vi "Sequence Init.vi"(8 "error in (no error)":errorcluster, 11 "CAP-USB-1 in":refnum<class "CAP-USB-1.lvclass">) -> (0 "error out":errorcluster, 3 "CAP-USB-1 out":refnum<class "CAP-USB-1.lvclass">)   [LabVIEW 2014, in "CAP-USB-1.lvlib" / "CAP-USB-1.lvclass"]
doc: "Envia el codigo de inicializacion para el funcionamiento en modo Sequence"
uses:
  CAP-USB-1.lvclass
  CAP-USB-1.lvclass/CAP-USB-1.ctl
  API/CAP-USB/CAP-USB.lvlib
  DriverMasterSync/build/DriverMasterSync.lvlibp/Modules/HAL/DriverMasterSync/DriverMasterSyncClass/DriverMasterSync.lvclass
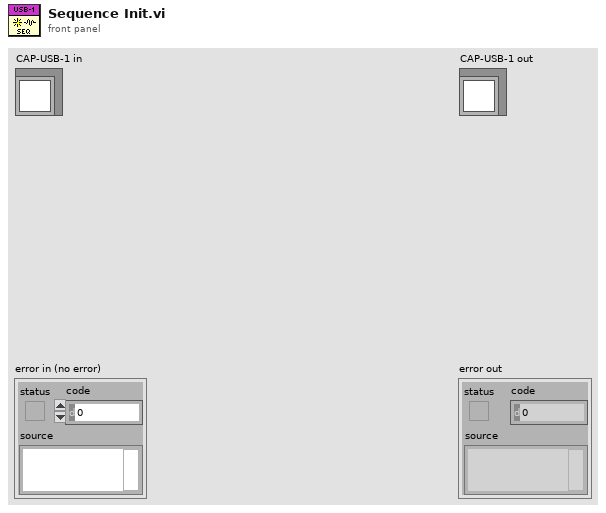
[diagram p1: front panel]
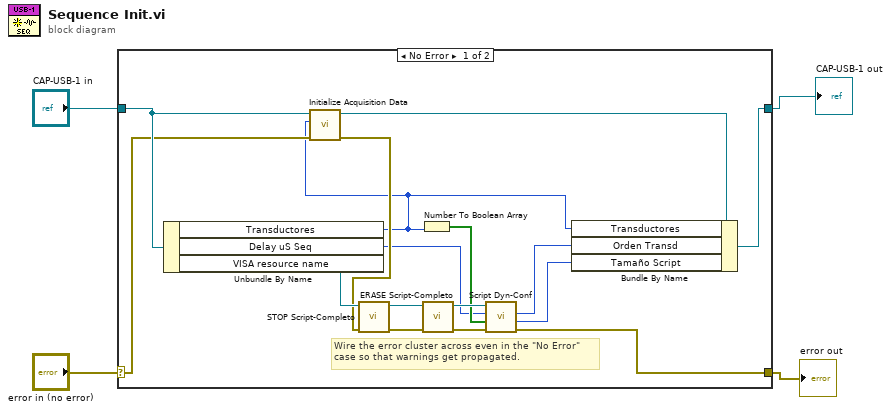
[diagram p0: block diagram]
diagram:
  n1 = case shown="No Error" "error in (no error)" {
    selector: "error in (no error)" -> [w8 w22]
    tunnel: [w16 w22] -> w1
    tunnel: [w11 w21] -> w2
    tunnel: "CAP-USB-1 in" -> [w10 w21]
    frame No Error {
      # "Wire the error cluster across even in the \"No Error\"\ncase so that warnings get propagated."
      n2 = Unbundle By Name(w10) -> ("Transductores"=w5:u64, "Delay uS Seq"=w6:i32, "VISA resource name"=w14:refnum<visa-resource-name>)
      n3 = call "Initialize Acquisition Data.vi"("error in (no error)"=w8, "Channel Mask"=w5, "DriverMasterSync in"=w10) -> ("error out"=w7:errorcluster, "DriverMasterSync out"=w9:refnum<class "CAP-USB-1.lvclass">)  [unwired: 7 in]
      n4 = call "STOP Script-Completo.vi"("error in (no error)"=w7, "VISA resource name"=w14) -> ("error out"=w19:errorcluster, "VISA resource name out"=w20:refnum<visa-resource-name>)  [unwired: 8 in]
      n5 = Number To Boolean Array(number=w5) -> (Boolean array=w15:bool[])
      n6 = call "ERASE Script-Completo.vi"("error in (no error)"=w19, "VISA resource name"=w20) -> ("error out"=w17:errorcluster, "VISA resource name out"=w18:refnum<visa-resource-name>)  [unwired: 8 in]
      n7 = call "Script Dyn-Conf.vi"("error in (no error)"=w17, "TDX"=w15, "DelayuS"=w6, "VISA resource name IN"=w18) -> ("error out"=w16:errorcluster, "Tamaño Script"=w13:i32, "Orden Transd"=w12:u64)  [unwired: 2 in, 1 out]
      n8 = Bundle By Name(cluster=w9, "Transductores"=w5, "Orden Transd"=w12, "Tamaño Script"=w13) -> (w11:refnum<class "CAP-USB-1.lvclass">)
    }
    frame Error {
    }
  }
  "error out" <- w1
  "CAP-USB-1 out" <- w2
